vi "Test DAQ Backpressure.vi"() -> ()   [LabVIEW 2021]
uses:
  ChannelCommon/typedef/FIFO Config.ctl
  ChannelCommon/ChannelCommon.lvlib
  CIFChannels/Typedef/Direction.ctl
  CIFChannels/CIFChannels.lvclass
  CIF_CIPC_Fifo_DAQ.lvclass
  ChannelCommon/typedef/TimeStamps.ctl
  ChannelCommon/typedef/Datatype Waveform.ctl
  ChannelCommon/typedef/New FIFO Instance Configuration.ctl
panel:
  out "status":string
  out "pass":bool
  out "error out":errorcluster
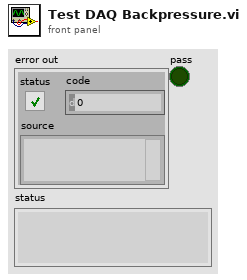
[diagram p1: front panel]
types:
  T1 = typedef "CIFChannels.lvclass/Direction.ctl" = enum16{"Publisher", "Subscriber"}
  T2 = typedef "ChannelCommon.lvlib/New FIFO Instance Configuration.ctl" = cluster{"Backpressure":bool, "Bytes/Message Override":u32, "Messages/FIFO Override":u32, "Custom Data":u8[]}
  T3 = typedef "ChannelCommon.lvlib/TimeStamps.ctl" = cluster{"ClockID":u8, "T0":i64, "T_Out":i64}
  T4 = typedef "ChannelCommon.lvlib/FIFO Config.ctl" = cluster{"Max Bytes/Msg":u64, "Max Msg/FIFO":u64, "Flags":u64}
  T5 = typedef "ChannelCommon.lvlib/Datatype Waveform.ctl" = cluster{"Measurement":dbl[], "dT":dbl, "Timestamp":i64}
  T6 = typedef "ChannelCommon.lvlib/New FIFO Instance Response.ctl" = cluster{"Publisher":string, "Custom Data":u8[]}
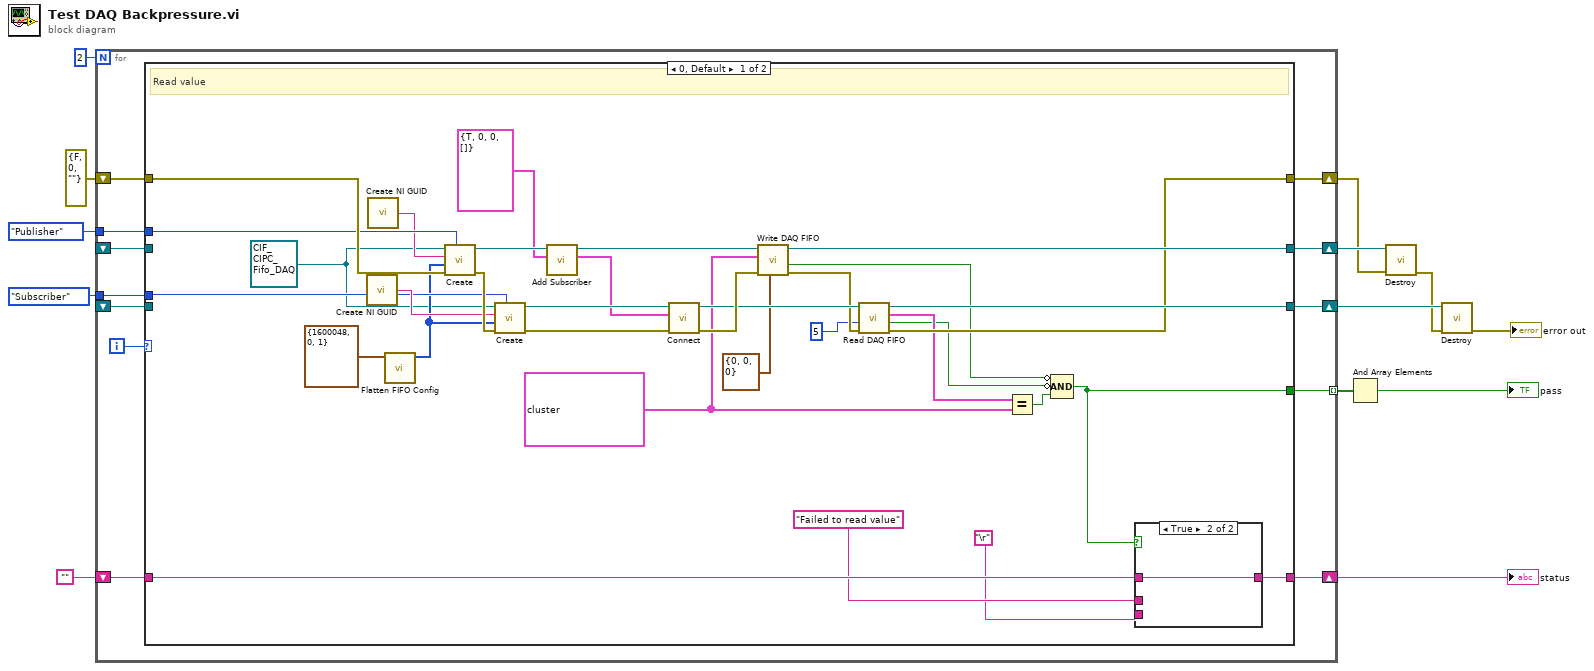
[diagram p0: block diagram]
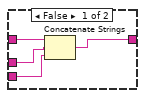
[diagram p2: hidden frame]
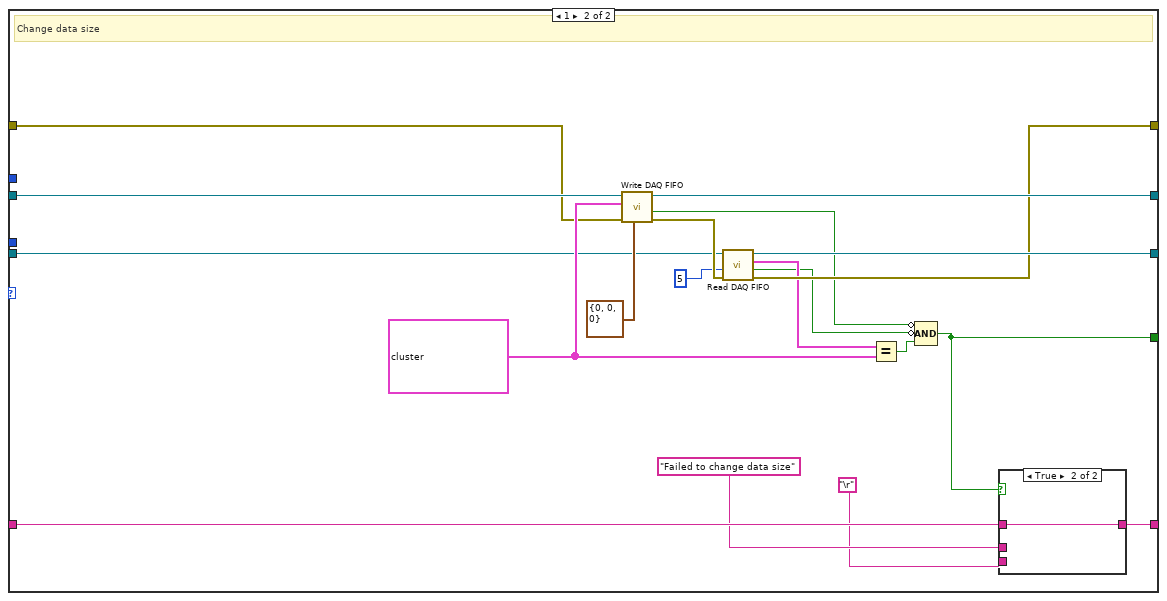
[diagram p3: hidden frame]
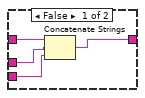
[diagram p4: hidden frame]
diagram:
  n1 = for {
    N: 2 -> [_]
    tunnel: [w25] -> w13 mode=indexing
    shift-right: [w23] -> w3
    shift-left: errorcluster {"status"=FALSE, "code"=0, "source"=""} ("error out") -> [w24]
    shift-right: [w20] -> w9
    shift-left: "" -> [w21]
    tunnel: Direction."Subscriber" ("Direction") -> [w19]
    tunnel: Direction."Publisher" ("Direction") -> [w18]
    shift-right: [w17] -> w5
    shift-left: _ -> [w15]
    shift-right: [w16] -> w4
    shift-left: _ -> [w14]
    i -> [w22]
    n2 = case shown="0, Default" w22 {
      tunnel: [w53 w77] -> w25
      tunnel: w24 -> [w51 w64]
      tunnel: [w39 w74] -> w23
      tunnel: w21 -> [w58 w82]
      tunnel: [w57 w81] -> w20
      tunnel: w19 -> [w49 _]
      tunnel: w18 -> [w48 _]
      tunnel: [w40 w75] -> w17
      tunnel: [w42 w76] -> w16
      tunnel: w14 -> [_ w66]
      tunnel: w15 -> [_ w65]
      frame 0, Default {
        w30 = T5[] [{"Measurement"=array[100000 elements], "dT"=2.0, "Timestamp"=3}] ("Data In")
        w32 = refnum<class "CIF_CIPC_Fifo_DAQ.lvclass"> refnum ("CIF_CIPC_Fifo_U8.lvclass")
        # "Read value"
        n3 = call <vilib>:"Create NI GUID.vi"() -> ("NI GUID"=w50:string)
        n4 = call <vilib>:"Create NI GUID.vi"() -> ("NI GUID"=w46:string)
        n5 = call "Flatten FIFO Config.vi"("FIFO Config in"=T4 {"Max Bytes/Msg"=1600048, "Max Msg/FIFO"=0, "Flags"=1}) -> ("Flattened FIFO Config"=w33:u8[])  [unwired: 10 in]
        n6 = call-dynamic "Create.vi"("Direction"=w48, "error in (no error)"=w51, "Custom Config Data"=w33, "Name"=w46, "CIFFIFO in"=w32) -> ("error out"=w52:errorcluster, "CIFFIFO out"=w29:refnum<class "CIF_CIPC_Fifo_DAQ.lvclass">)  [unwired: 5 in]
        n7 = call-dynamic "Create.vi"("Direction"=w49, "error in (no error)"=w52, "Custom Config Data"=w33, "Name"=w50, "CIFFIFO in"=w32) -> ("error out"=w45:errorcluster, "CIFFIFO out"=w44:refnum<class "CIF_CIPC_Fifo_DAQ.lvclass">)  [unwired: 5 in]
        n8 = call-dynamic "Add Subscriber.vi"("New FIFO Instance Config"=T2 {"Backpressure"=TRUE, "Bytes/Message Override"=0, "Messages/FIFO Override"=0, "Custom Data"=[]}, "CIF_CIPC_Chn in"=w29) -> ("New FIFO Instance"=w28:T6, "CIF_CIPC_Chn out"=w27:refnum<class "CIF_CIPC_Fifo_DAQ.lvclass">)  [unwired: 7 in, 1 out]
        n9 = call-dynamic "Connect.vi"("error in (no error)"=w45, "Connection"=w28, "CIFTag in"=w44) -> ("error out"=w43:errorcluster, "CIFTag out"=w41:refnum<class "CIF_CIPC_Fifo_DAQ.lvclass">)  [unwired: 7 in]
        n10 = call-dynamic "Write DAQ FIFO.vi"("FIFO Timestamps"=T3 {"ClockID"=0, "T0"=0, "T_Out"=0}, "error in (no error)"=w43, "Data In"=w30, "CIFFIFO in"=w27) -> ("error out"=w38:errorcluster, "timed out?"=w37:bool, "CIFFIFO out"=w42:refnum<class "CIF_CIPC_Fifo_DAQ.lvclass">)  [unwired: 4 in, 1 out]
        n11 = call-dynamic "Read DAQ FIFO.vi"("error in (no error)"=w38, "Timeout (ms)"=5, "CIFFIFO in"=w41) -> ("error out"=w39:errorcluster, "timed out?"=w35:bool, "Data Out"=w36:T5[], "CIFFIFO out"=w40:refnum<class "CIF_CIPC_Fifo_DAQ.lvclass">)  [unwired: 4 in, 1 out]
        n12 = Equal?(x=w36, y=w30) -> (x = y?=w54:bool)
        n13 = Compound Arithmetic op=AND(invert w37, invert w35, w54) -> (w53:bool)
        n14 = case shown="True" w53 {
          tunnel: w58 -> [w62 w63]
          tunnel: [w59 w63] -> w57
          tunnel: "Failed to read value" -> [w61 _]
          tunnel: "\r" -> [w60 _]
          frame False {
            n15 = Concatenate Strings(w62, w61, w60) -> (w59:string)
          }
          frame True {
          }
        }
      }
      frame 1 {
        w67 = T5[] [{"Measurement"=array[100000 elements], "dT"=2.0, "Timestamp"=3}, {"Measurement"=array[100000 elements], "dT"=0.0, "Timestamp"=0}] ("Data In")
        # "Change data size"
        n16 = call-dynamic "Write DAQ FIFO.vi"("FIFO Timestamps"=T3 {"ClockID"=0, "T0"=0, "T_Out"=0}, "error in (no error)"=w64, "Data In"=w67, "CIFFIFO in"=w66) -> ("error out"=w73:errorcluster, "timed out?"=w72:bool, "CIFFIFO out"=w76:refnum<class "CIF_CIPC_Fifo_DAQ.lvclass">)  [unwired: 4 in, 1 out]
        n17 = call-dynamic "Read DAQ FIFO.vi"("error in (no error)"=w73, "Timeout (ms)"=5, "CIFFIFO in"=w65) -> ("error out"=w74:errorcluster, "timed out?"=w70:bool, "Data Out"=w71:T5[], "CIFFIFO out"=w75:refnum<class "CIF_CIPC_Fifo_DAQ.lvclass">)  [unwired: 4 in, 1 out]
        n18 = Equal?(x=w71, y=w67) -> (x = y?=w78:bool)
        n19 = Compound Arithmetic op=AND(invert w72, invert w70, w78) -> (w77:bool)
        n20 = case shown="True" w77 {
          tunnel: w82 -> [w86 w87]
          tunnel: [w83 w87] -> w81
          tunnel: "Failed to change data size" -> [w85 _]
          tunnel: "\r" -> [w84 _]
          frame False {
            n21 = Concatenate Strings(w86, w85, w84) -> (w83:string)
          }
          frame True {
          }
        }
      }
    }
  }
  "status" <- w9
  n22 = And Array Elements(Boolean array=w13) -> (logical AND=→"pass":bool)
  n23 = call-dynamic "Destroy.vi"("error in (no error)"=w3, "CIFTag in"=w4) -> ("error out"=w2:errorcluster)  [unwired: 8 in, 1 out]
  n24 = call-dynamic "Destroy.vi"("error in (no error)"=w2, "CIFTag in"=w5) -> ("error out"=→"error out":errorcluster)  [unwired: 8 in, 1 out]
